vi "Unregister with Manager.vi"(8 "error in (no error)":errorcluster, 10 "Unregister Channels":string[](array[string]), 11 "CIFCorePlugin in":refnum<class "CIFCorePlugin.lvclass">) -> (0 "error out":errorcluster, 3 "CIFCorePlugin out":refnum<class "CIFCorePlugin.lvclass">)   [LabVIEW 2021, in "CIFCorePlugin.lvclass"]
uses:
  CIFCorePlugin.lvclass
  CIFCorePlugin.lvclass/CIFCorePlugin.ctl
  CIFPluginManager/CIFPluginManager/gRPC/CIF_Manager_Client_Wrapper/CIFManagerClientWrapper.lvlib
  CIFPluginManager/CIFPluginManager/gRPC/CIF_Manager_client/RPC Messages/cif_manager_UnregisterData.ctl
  CIFPluginManager/CIFPluginManager/gRPC/CIF_Manager_client/CIF_Manager_client.lvlib
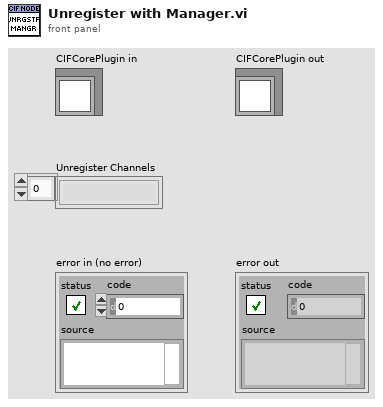
[diagram p1: front panel]
types:
  T1 = typedef "grpc-lvsupport-release.lvlib/grpcId.ctl" = u64
  T2 = typedef "CIF_Manager_client.lvlib/cif_manager_UnregisterData.ctl" = cluster{"plugin_name":string, "unregister_channels":string[]}
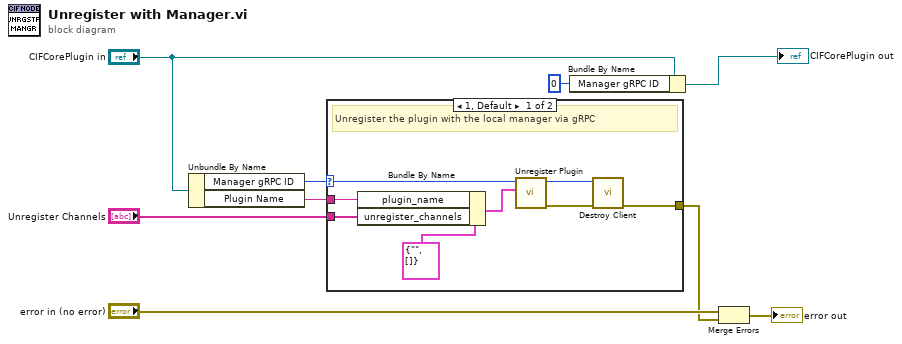
[diagram p0: block diagram]
diagram:
  n1 = Unbundle By Name("CIFCorePlugin in") -> ("Manager gRPC ID"=w9:T1, "Plugin Name"=w2:string)
  n2 = case shown="1, Default" w9 {
    selector: w9 -> [w17 _]
    tunnel: [w14 _] -> w5
    tunnel: w2 -> [w12 _]
    tunnel: "Unregister Channels" -> [w10 _]
    frame 1, Default {
      # "Unregister the plugin with the local manager via gRPC"
      n3 = Bundle By Name(cluster=T2 {"plugin_name"="", "unregister_channels"=[]} ("Unregister"), "plugin_name"=w12, "unregister_channels"=w10) -> (w11:T2)
      n4 = call "Unregister Plugin.vi"("Unregister"=w11, "gRPC ID in"=w17) -> ("error out"=w15:errorcluster, "gRPC ID out"=w16:T1)  [unwired: 8 in]
      n5 = call "Destroy Client.vi"("error in"=w15, "gRPC ID"=w16) -> ("error out"=w14:errorcluster)  [unwired: 9 in]
    }
    frame 0 {
      # "During testing manager may not be present.  No valid handle for gRPC Client."
    }
  }
  n6 = Bundle By Name(cluster="CIFCorePlugin in", "Manager gRPC ID"=u64 0) -> (→"CIFCorePlugin out":refnum<class "CIFCorePlugin.lvclass">)
  n7 = Merge Errors("error in (no error)", w5) -> (→"error out":errorcluster)
